vi "PodStateComms.vi"(8 "error in":errorcluster, 11 "Pod State":T1) -> (0 "error out":errorcluster)   [LabVIEW 2017]
uses:
  Type Defs/PodState.ctl
panel:
  out "Buttons":bool[](array[boolean])
  out "Pod State":bool[](array[boolean])
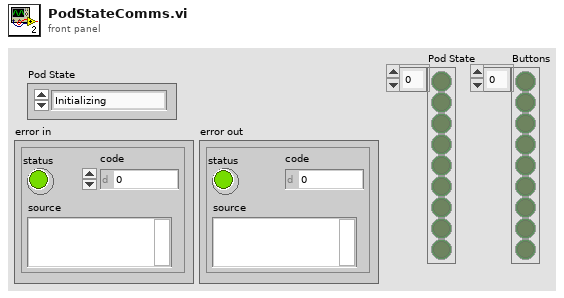
[diagram p1: front panel]
types:
  T1 = typedef "PodState.ctl" = enum16{"Initializing", "Pre-flight Testing", "Ready", "Pushing", "Coast", "Braking", "Post-flight", "Fault"}
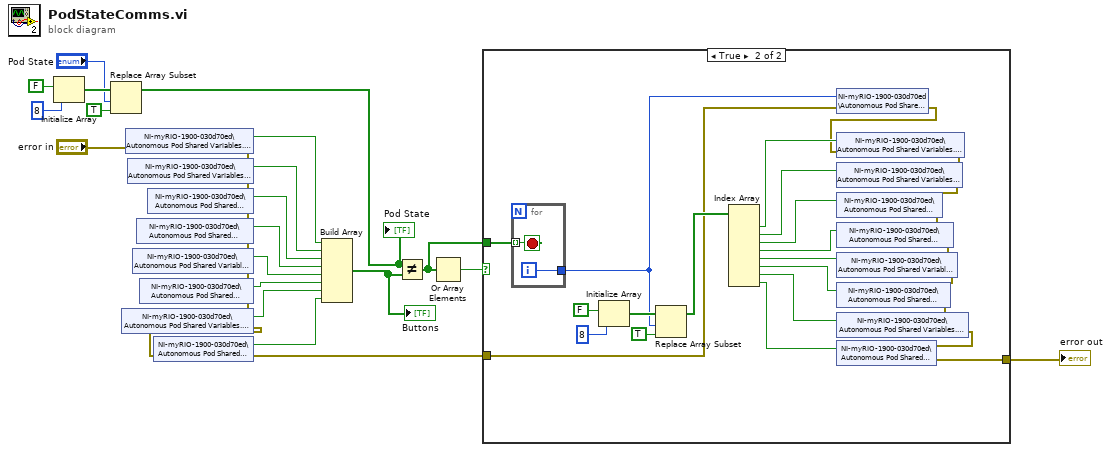
[diagram p0: block diagram]
diagram:
  n1 = Initialize Array(FALSE ("State:Initializing"), 8 ("dimension size")) -> (w12:bool[])
  n2 = Replace Array Subset(array=w12, new element=TRUE ("new element/subarray"), index="Pod State") -> (w10:bool[])
  "Pod State" <- w10
  n3 = shared-variable "NI-myRIO-1900-030d70ed\\Autonomous Pod Shared Variables.lvlib\\State:Initializing"(error in="error in") -> (w4:bool, error out=w27:errorcluster)
  n4 = shared-variable "NI-myRIO-1900-030d70ed\\Autonomous Pod Shared Variables.lvlib\\State:Pre-Flight"(error in=w27) -> (w5:bool, error out=w26:errorcluster)
  n5 = shared-variable "NI-myRIO-1900-030d70ed\\Autonomous Pod Shared Variables.lvlib\\State:Ready"(error in=w26) -> (w20:bool, error out=w25:errorcluster)
  n6 = shared-variable "NI-myRIO-1900-030d70ed\\Autonomous Pod Shared Variables.lvlib\\State:Pushing"(error in=w25) -> (w19:bool, error out=w24:errorcluster)
  n7 = shared-variable "NI-myRIO-1900-030d70ed\\Autonomous Pod Shared Variables.lvlib\\State:Coasting"(error in=w24) -> (w18:bool, error out=w23:errorcluster)
  n8 = shared-variable "NI-myRIO-1900-030d70ed\\Autonomous Pod Shared Variables.lvlib\\State:Braking"(error in=w23) -> (w17:bool, error out=w22:errorcluster)
  n9 = shared-variable "NI-myRIO-1900-030d70ed\\Autonomous Pod Shared Variables.lvlib\\State:Post-Flight"(error in=w22) -> (w16:bool, error out=w2:errorcluster)
  n10 = shared-variable "NI-myRIO-1900-030d70ed\\Autonomous Pod Shared Variables.lvlib\\State:Fault"(error in=w2) -> (w15:bool, error out=w9:errorcluster)
  n11 = Build Array(w4, w5, w20, w19, w18, w17, w16, w15) -> (w3:bool[])
  "Buttons" <- w3
  n12 = Not Equal?(x=w10, y=w3) -> (x != y?=w7:bool[])
  n13 = Or Array Elements(Boolean array=w7) -> (logical OR=w8:bool)
  n14 = case shown="True" w8 {
    tunnel: w9 -> [w28 w33]
    tunnel: w7 -> [_ w47]
    tunnel: [w28 w34] -> w6
    frame False {
    }
    frame True {
      n15 = for {
        tunnel: w47 -> [w55] mode=indexing
        tunnel: [w54] -> w32
        i -> [w54]
        stop <- w55 stop-if-true
      }
      n16 = Initialize Array(FALSE ("State:Initializing"), 8 ("dimension size")) -> (w45:bool[])
      n17 = Replace Array Subset(array=w45, new element=TRUE ("new element/subarray"), index=w32) -> (w42:bool[])
      n18 = Index Array(array=w42) -> (element #1=w41:bool, element #2=w40:bool, element #3=w39:bool, element #4=w38:bool, element #5=w37:bool, element #6=w36:bool, element #7=w35:bool, element #8=w30:bool)  [unwired: 8 in]
      n19 = shared-variable "NI-myRIO-1900-030d70ed\\Autonomous Pod Shared Variables.lvlib\\PodState"(w32, error in=w33) -> (error out=w31:errorcluster)
      n20 = shared-variable "NI-myRIO-1900-030d70ed\\Autonomous Pod Shared Variables.lvlib\\State:Initializing"(w41, error in=w31) -> (error out=w48:errorcluster)
      n21 = shared-variable "NI-myRIO-1900-030d70ed\\Autonomous Pod Shared Variables.lvlib\\State:Pre-Flight"(w40, error in=w48) -> (error out=w49:errorcluster)
      n22 = shared-variable "NI-myRIO-1900-030d70ed\\Autonomous Pod Shared Variables.lvlib\\State:Ready"(w39, error in=w49) -> (error out=w50:errorcluster)
      n23 = shared-variable "NI-myRIO-1900-030d70ed\\Autonomous Pod Shared Variables.lvlib\\State:Pushing"(w38, error in=w50) -> (error out=w51:errorcluster)
      n24 = shared-variable "NI-myRIO-1900-030d70ed\\Autonomous Pod Shared Variables.lvlib\\State:Coasting"(w37, error in=w51) -> (error out=w52:errorcluster)
      n25 = shared-variable "NI-myRIO-1900-030d70ed\\Autonomous Pod Shared Variables.lvlib\\State:Braking"(w36, error in=w52) -> (error out=w53:errorcluster)
      n26 = shared-variable "NI-myRIO-1900-030d70ed\\Autonomous Pod Shared Variables.lvlib\\State:Post-Flight"(w35, error in=w53) -> (error out=w29:errorcluster)
      n27 = shared-variable "NI-myRIO-1900-030d70ed\\Autonomous Pod Shared Variables.lvlib\\State:Fault"(w30, error in=w29) -> (error out=w34:errorcluster)
    }
  }
  "error out" <- w6
